vi "WinAPI.SetTopMost.vi"(8 "error in (no error)":errorcluster, 11 "hWnd":u64) -> (0 "error out":errorcluster)   [LabVIEW 2013, in "ToolbarMenu.lvlib"]
uses:
  ToolbarMenu.lvlib
  <vilib>/Utility/error.llb/Error Cluster From Error Code.vi
  <vilib>/ErrorRing/Error Ring.xnode
  user32.dll
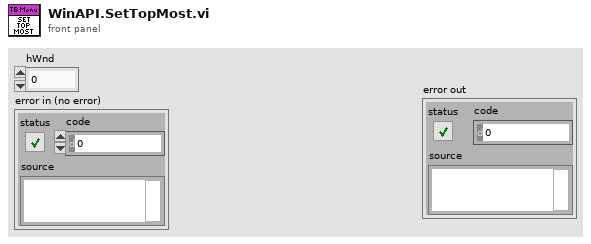
[diagram p1: front panel]
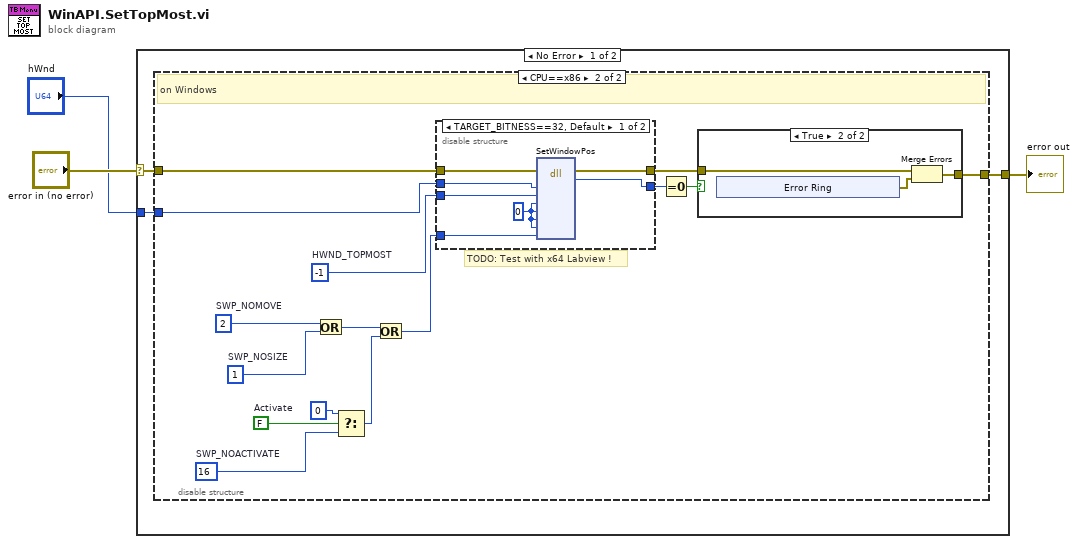
[diagram p0: block diagram]
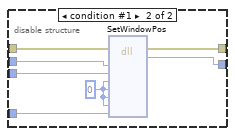
[diagram p3: hidden frame]
diagram:
  n1 = case shown="No Error" "error in (no error)" {
    selector: "error in (no error)" -> [w5 w46]
    tunnel: [w6 w46] -> w3
    tunnel: "hWnd" -> [w4 _]
    frame No Error {
      n2 = disable-structure shown="CPU==x86" {
        disable-tunnel: [w7 w22] -> w6
        disable-tunnel: w5 -> [w7 w21]
        disable-tunnel: w4 -> [_ w8]
        frame condition #0 {
          # "Ignore TopMost"
        }
        frame condition #1 (active) {
          w10 = FALSE  # Activate
          w11 = u32 2  # SWP_NOMOVE
          w12 = u32 1  # SWP_NOSIZE
          w13 = u32 16  # SWP_NOACTIVATE
          w20 = -1  # HWND_TOPMOST
          # "TODO: Test with x64 Labview !"
          # "on Windows"
          n3 = Or(x=w11, y=w12) -> (x .or. y?=w16:u32)
          n4 = Select(t=u32 0, s=w10, f=w13) -> (s? t:f=w15:u32)
          n5 = Or(x=w16, y=w15) -> (x .or. y?=w9:u32)
          n6 = disable-structure shown="TARGET_BITNESS==32, Default" {
            disable-tunnel: w20 -> [w29 w31]
            disable-tunnel: w8 -> [w28 w32]
            disable-tunnel: w21 -> [w27 w35]
            disable-tunnel: [w26 w33] -> w19
            disable-tunnel: [w24 w34] -> w18
            disable-tunnel: w9 -> [w23 w30]
            frame condition #0 (active) {
              w25 = 0
              n7 = dll-call lib="USER32.DLL" fn="SetWindowPos" label="SetWindowPosx86"(error in=w27, "hWnd"=w28, "hWndInsertAfter"=w29, "left"=w25, "top"=w25, "width"=w25, "height"=w25, "fuFlags"=w23) -> (error out=w26:errorcluster, "error"=w24:i32)  [unwired: 8 in, 2 out]
            }
            frame condition #1 {
              w36 = 0
              n8 = dll-call lib="USER32.DLL" fn="SetWindowPos" label="SetWindowPosx64"(error in=w35, "hWnd"=w32, "hWndInsertAfter"=w31, "left"=w36, "top"=w36, "width"=w36, "height"=w36, "fuFlags"=w30) -> (error out=w33:errorcluster, "error"=w34:i64)  [unwired: 8 in, 2 out]
            }
          }
          n9 = Equal To 0?(x=w18) -> (x = 0?=w17:bool)
          n10 = case shown="True" w17 {
            tunnel: w19 -> [w37 w39]
            tunnel: [w37 w38] -> w22
            frame False {
            }
            frame True {
              n11 = xnode "Error Ring"() -> ("error out"=w40:errorcluster)
              n12 = Merge Errors(w39, w40) -> (w38:errorcluster)
            }
          }
        }
      }
    }
    frame Error {
    }
  }
  "error out" <- w3
